vi "Dispose Test Client.vi"(8 "error in (no error)":errorcluster, 11 "Test Redis Client in":refnum<class "Test Redis Client.lvclass">) -> (0 "error out":errorcluster)   [LabVIEW 2019, in "Test Redis Client for LabVIEW.lvlib" / "Test Redis Client.lvclass"]
uses:
  Test Redis Client.lvclass
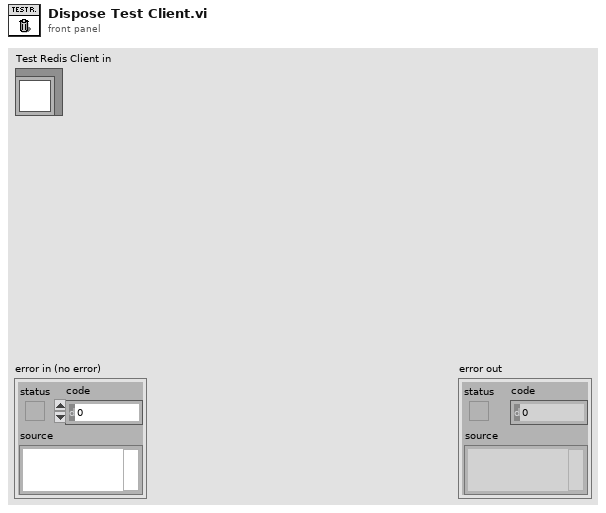
[diagram p1: front panel]
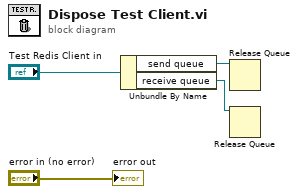
[diagram p0: block diagram]
diagram:
  n1 = Unbundle By Name("Test Redis Client in") -> ("send queue"=w2:refnum<queue>, "receive queue"=w1:refnum<queue>)
  n2 = Release Queue(queue=w2) -> ()  [unwired: 2 in, 3 out]
  n3 = Release Queue(queue=w1) -> ()  [unwired: 2 in, 3 out]
  "error out" <- "error in (no error)"
